vi "PreLoop.vi"(6 "Error":errorcluster, 7 "Actor":refnum<class "Actor Layer.lvclass">) -> (5 "Actor":refnum<class "Actor Layer.lvclass">)   [LabVIEW 2020, in "_Template.lvlib" / "{{Actor}}.lvlib" / "Actor Layer.lvclass"]
uses:
  Actor Layer.lvclass
  Actor Layer.lvclass/Actor Layer.ctl
  C:/Users/nathan.davis/Desktop/personal/jettl-harness/repos/jettl/src/jettl Tools/_Template/{{Actor}}/Actor Layer/Actor Layer.lvclass
  C:/Users/nathan.davis/Desktop/personal/jettl-harness/repos/jettl/src/jettl Tools/_Template/{{Msg}}/Actor Msg/Actor Msg.lvclass
  C:/Users/nathan.davis/Desktop/personal/jettl-harness/repos/jettl/src/jettl/jettl/Actor Layer/Actor Layer.lvclass
  jettl/jettl/Actor Layer/Actor Layer.lvclass
panel:
  # "This front panel should not be manipulated."
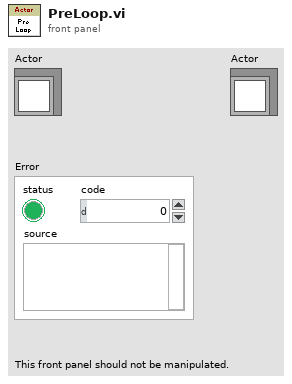
[diagram p1: front panel]
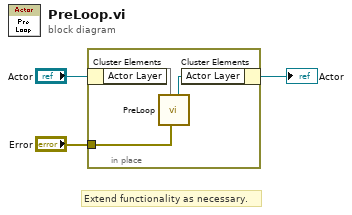
[diagram p0: block diagram]
diagram:
  # "Extend functionality as necessary."
  n1 = in-place {
    in-place-border: "Error" -> [w4]
    n2 = in-place-cluster #1("Actor") -> ("Actor Layer"=w6)
    n3 = call-dynamic "PreLoop.vi"("Error"=w4, "Actor"=w6) -> ("Actor"=w5:refnum<class "Actor Layer.lvclass">)  [unwired: 8 in, 1 out]
    n4 = in-place-cluster #1("Actor Layer"=w5) -> (→"Actor":refnum<class "Actor Layer.lvclass">)
  }
